vi "Get Plugin Summary Info.vi"(11 "CIF_UI in":refnum<class "CIF_UI.lvclass">) -> (3 "Plugin Summary Info":T1[](array[typedef]))   [LabVIEW 2021, in "CIF_UI.lvclass"]
uses:
  CIF_UI.lvclass
  Typedef/Plugin Summary.ctl
  Typedef/Version.ctl
  CIF_UI.lvclass/CIF_UI.ctl
  3cb97bbe-ec67-4187-806b-96be001ee38f.vi
  <vilib>/Comparison/Less/Less Functor/Less Functor.lvclass
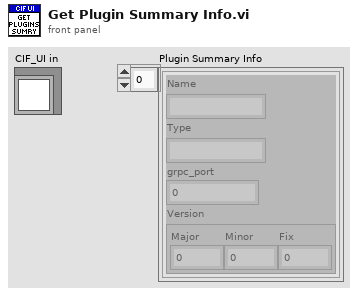
[diagram p1: front panel]
types:
  T1 = typedef "CIF_UI.lvclass/Plugin Summary.ctl" = cluster{"Name":string, "Type":string, "grpc_port":i32, "Version":T2}
  T2 = typedef "CIF_UI.lvclass/Version.ctl" = cluster{"Major":i32, "Minor":i32, "Fix":i32}
  T3 = typedef "CIF_UI.lvclass/Plugin Connection Map.ctl" = map{string, T4}
  T4 = typedef "CIF_UI.lvclass/Plugin Connections.ctl" = cluster{"gRPC ID":T5, "Plugin Info":T6}
  T5 = typedef "grpc-lvsupport-release.lvlib/grpcId.ctl" = u64
  T6 = typedef "CIF_UI.lvclass/PluginInfo.ctl" = cluster{"Name":string, "Type":string, "grpc_port":i32, "Version":T2, "Node Status":T7}
  T7 = typedef "CIFCoreCommon.lvlib/gRPC Reported Plugin Status.ctl" = cluster{"State":T8, "Timing Statistics (us)":T9, "FIFO Statistics (us)":T11, "error":T12, "Monitor Doubles":T13, "Monitor U64":T14, "Monitor I64":T15}
  T8 = typedef "CIFCoreCommon.lvlib/Plugin State.ctl" = enum32{"Null", "Creating", "Listening", "Running", "CleaningUp", "Destroying"}
  T9 = typedef "CIFCoreCommon.lvlib/Timing Statistics.ctl" = cluster{"Period":T10, "Wake Error":T10, "Execute":T10, "Housekeep":T10, "Idle":T10, "Cleanup":T10, "Custom 1 (custom units)":T10, "Custom 2 (custom units)":T10}
  T10 = typedef "CIFCoreCommon.lvlib/Timing Stats Base.ctl" = cluster{"Max":i64, "Avg":dbl, "Min":i64}
  T11 = typedef "CIFCoreCommon.lvlib/FIFO Statistics.ctl" = cluster{"From T0":T10, "From Previous Plugin":T10, "Output Error":T10}
  T12 = typedef "CIFCoreCommon.lvlib/Simple Error.ctl" = cluster{"status":bool, "code":i32}
  T13 = typedef "CIFCoreCommon.lvlib/Monitor Doubles.ctl" = cluster{"1":dbl, "2":dbl, "3":dbl, "4":dbl}
  T14 = typedef "CIFCoreCommon.lvlib/Monitor U64.ctl" = cluster{"1":u64, "2":u64, "3":u64, "4":u64}
  T15 = typedef "CIFCoreCommon.lvlib/Monitor I64.ctl" = cluster{"1":i64, "2":i64, "3":i64, "4":i64}
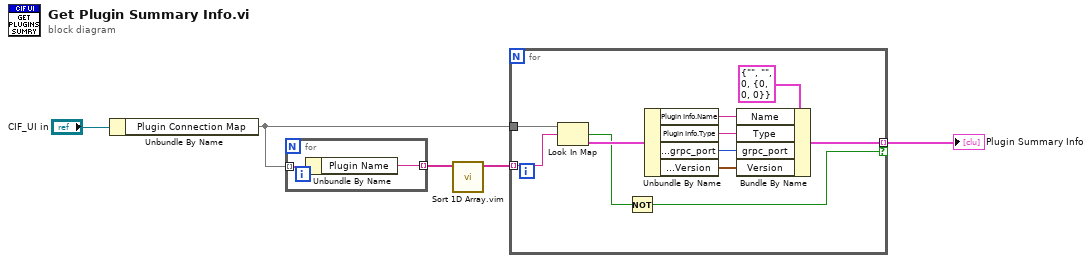
[diagram p0: block diagram]
diagram:
  n1 = Unbundle By Name("CIF_UI in") -> ("Plugin Connection Map"=w1:T3)
  n2 = for {
    tunnel: w1 -> [w6] mode=indexing
    tunnel: [w7] -> w3 mode=indexing
    n3 = Unbundle By Name(w6) -> ("Plugin Name"=w7:string)
  }
  n4 = call "Sort 1D Array.vim"("unsorted array"=w3) -> ("sorted array"=w2:string[])  [unwired: 10 in]
  n5 = for {
    tunnel: [w18] -> w5 mode=indexing if=w17
    tunnel: w2 -> [w11] mode=indexing
    tunnel: w1 -> [w8]
    n6 = Look In Map(map=w8, key=w11) -> (key not found?=w9:bool, value=w10:T4)  [unwired: 1 in]
    n7 = Not(x=w9) -> (.not. x?=w17:bool)
    n8 = Unbundle By Name(w10) -> ("Plugin Info.Name"=w15:string, "Plugin Info.Type"=w12:string, "Plugin Info.grpc_port"=w13:i32, "Plugin Info.Version"=w14:T2)
    n9 = Bundle By Name(cluster=T1 {"Name"="", "Type"="", "grpc_port"=0, "Version"={"Major"=0, "Minor"=0, "Fix"=0}} ("Plugin Summary"), "Name"=w15, "Type"=w12, "grpc_port"=w13, "Version"=w14) -> (w18:T1)
  }
  "Plugin Summary Info" <- w5
